vi "Init Logging.vi"(8 "error in (no error)":errorcluster, 11 "Server in":refnum<class "Server.lvclass">) -> (0 "error out":errorcluster, 3 "Server out":refnum<class "Server.lvclass">)   [LabVIEW 2020, in "HTTP Server.lvlib" / "Server.lvclass"]
uses:
  Server.lvclass
  Access Log Entry.ctl
  Server.lvclass/Server.ctl
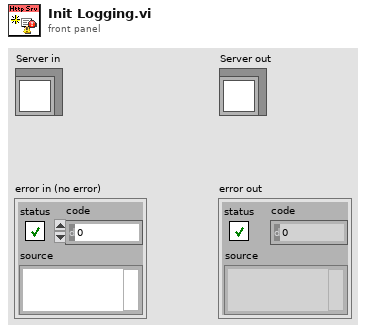
[diagram p1: front panel]
types:
  T1 = typedef "HTTP Server.lvlib/Server.lvclass/Access Log Entry.ctl" = cluster{"Time Stamp":timestamp, "Client":string, "Code":u16, "Info":string}
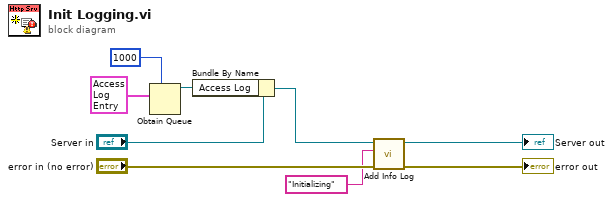
[diagram p0: block diagram]
diagram:
  n1 = Obtain Queue(max queue size (-1, unlimited)=1000, element data type=T1 {"Time Stamp"=timestamp(0 s since 1904-01-01), "Client"="", "Code"=0, "Info"=""} ("Log Entry")) -> (queue out=w6:refnum<queue>)  [unwired: 3 in, 2 out]
  n2 = Bundle By Name(cluster="Server in", "Access Log"=w6) -> (w4:refnum<class "Server.lvclass">)
  n3 = call "Add Info Log.vi"("error in (no error)"="error in (no error)", "Info"="Initializing", "Server in"=w4) -> ("error out"=→"error out":errorcluster, "Server out"=→"Server out":refnum<class "Server.lvclass">)  [unwired: 7 in]
